vi "Scripting_ChangeBaseClassInSubClass.vi"(0 "SubClass":refnum<vi>, 1 "NewBaseClass":path=path "C:/Projects/Base2_class/Base2.lvclass", 2 "GOOP4Style":bool, 5 "error in (no error)":errorcluster) -> (19 "error out":errorcluster={"status"=TRUE, "code"=1055, "source"="Property Node in Scripting_ConvertBaseClassToSubClass.vi"})   [LabVIEW 2012]
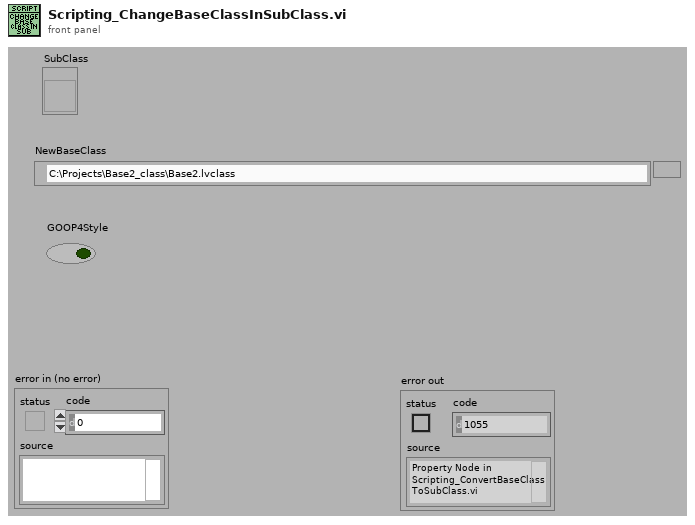
[diagram p1: front panel]
types:
  T1 = cluster{"NewBaseClass":refnum<vi>, "NewBaseClassPath":path, "SubClass":refnum<vi>, "NewBaseClassName":string, "AllBaseClassFiles":path[], "ClassVIs":refnum<vi>[], "CurrentBaseClassRef":refnum<vi>, "CurrentBaseClassPath":path, "CurrentRootBaseClassPath":path, "NewRootBaseClassPath":path}
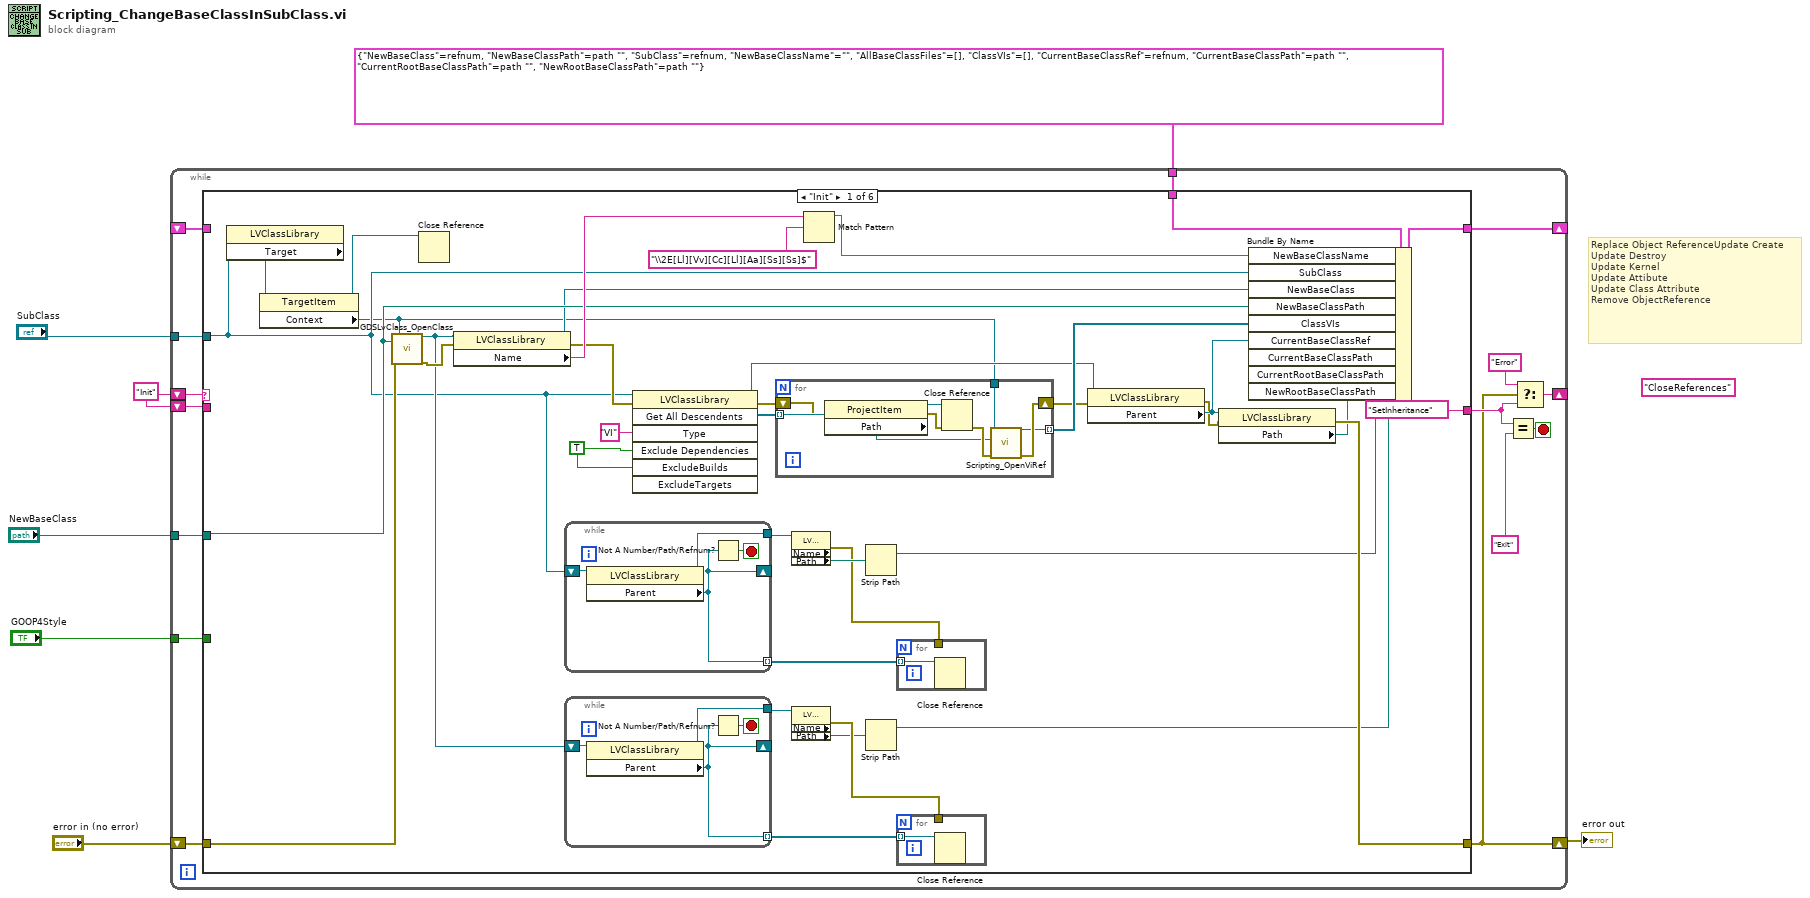
[diagram p0: block diagram]
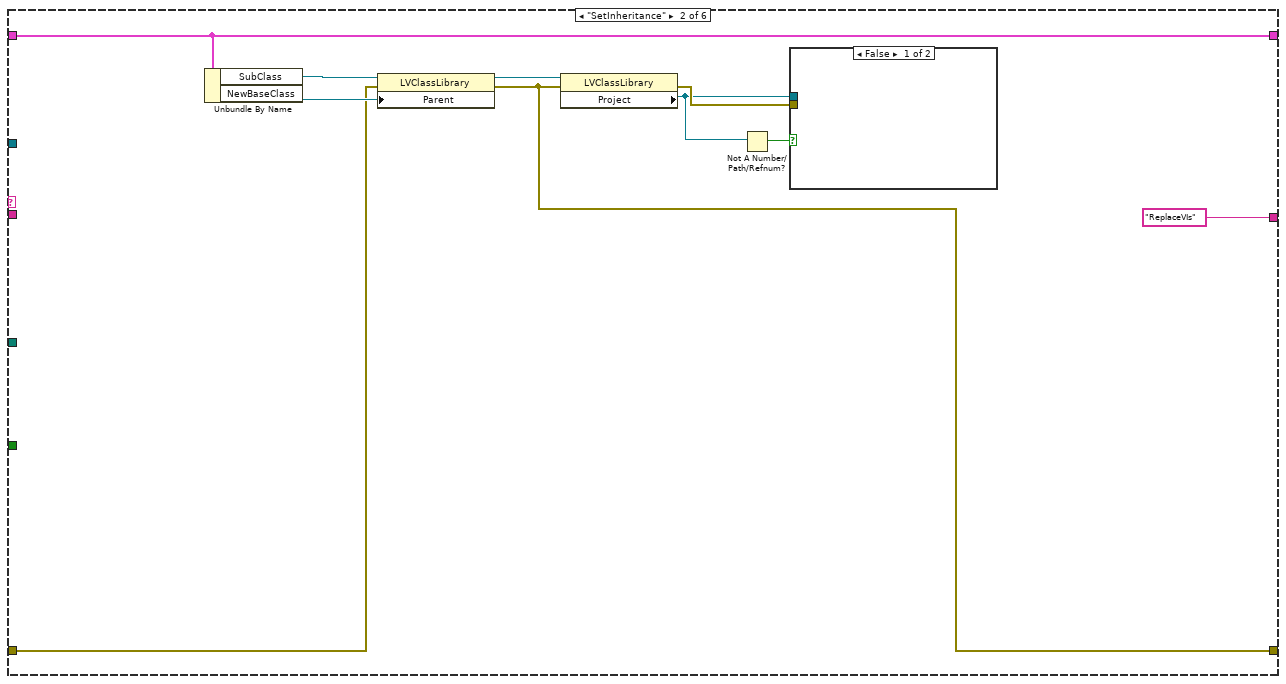
[diagram p2: hidden frame]
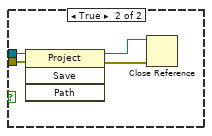
[diagram p3: hidden frame]
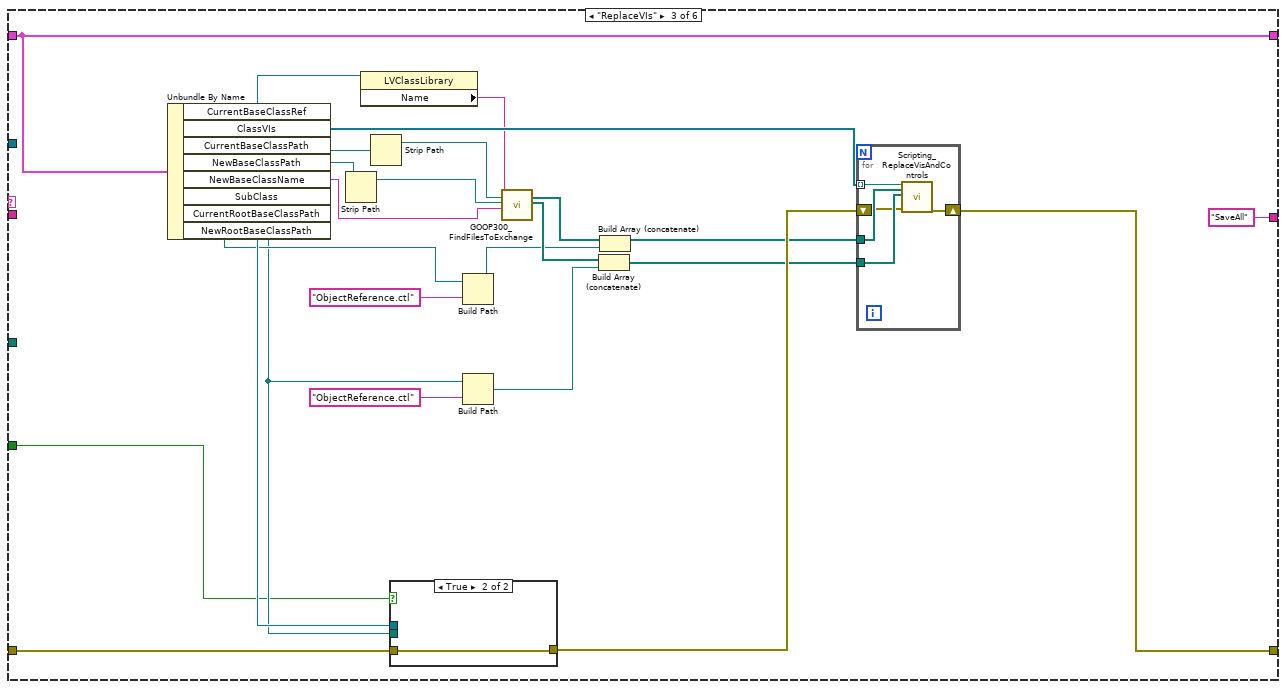
[diagram p4: hidden frame]
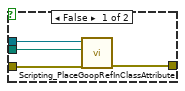
[diagram p5: hidden frame]
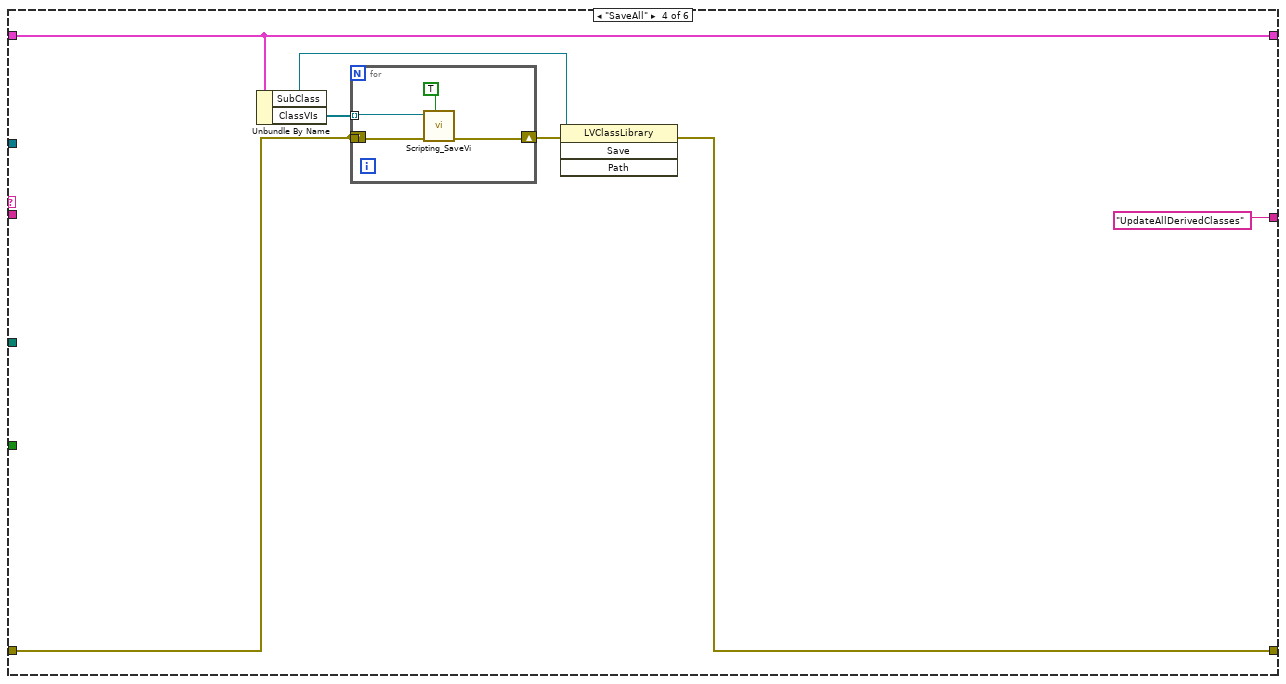
[diagram p6: hidden frame]
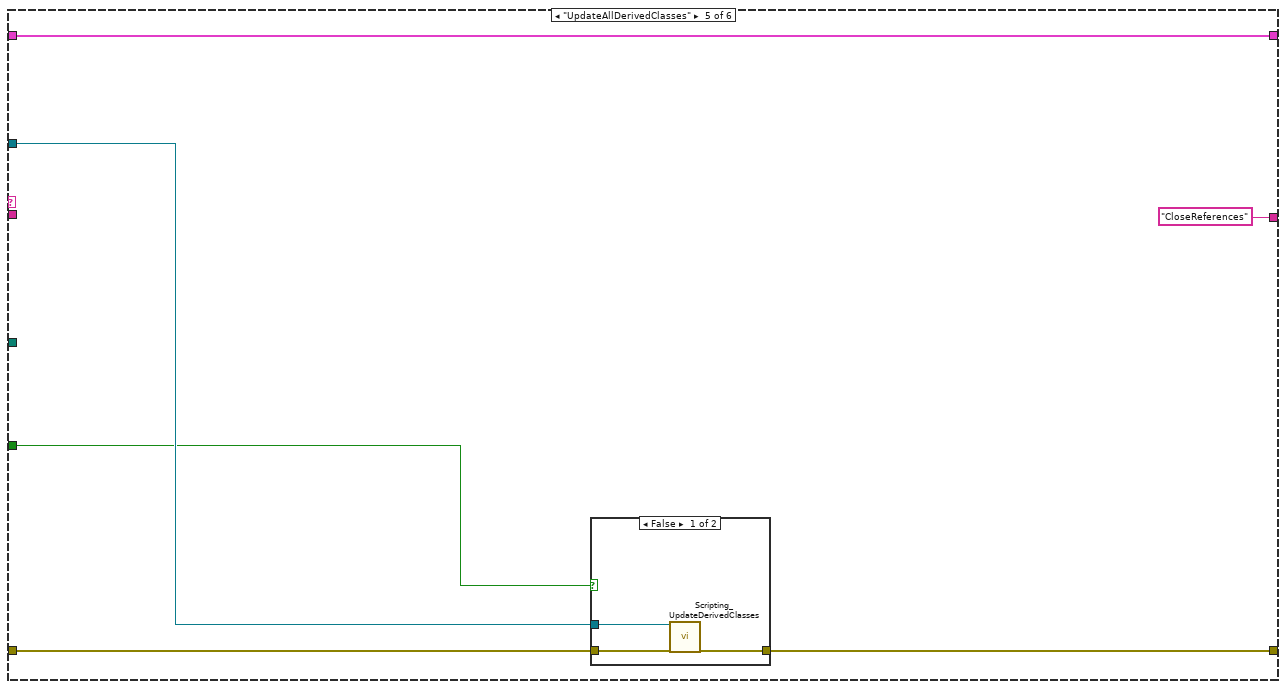
[diagram p7: hidden frame]
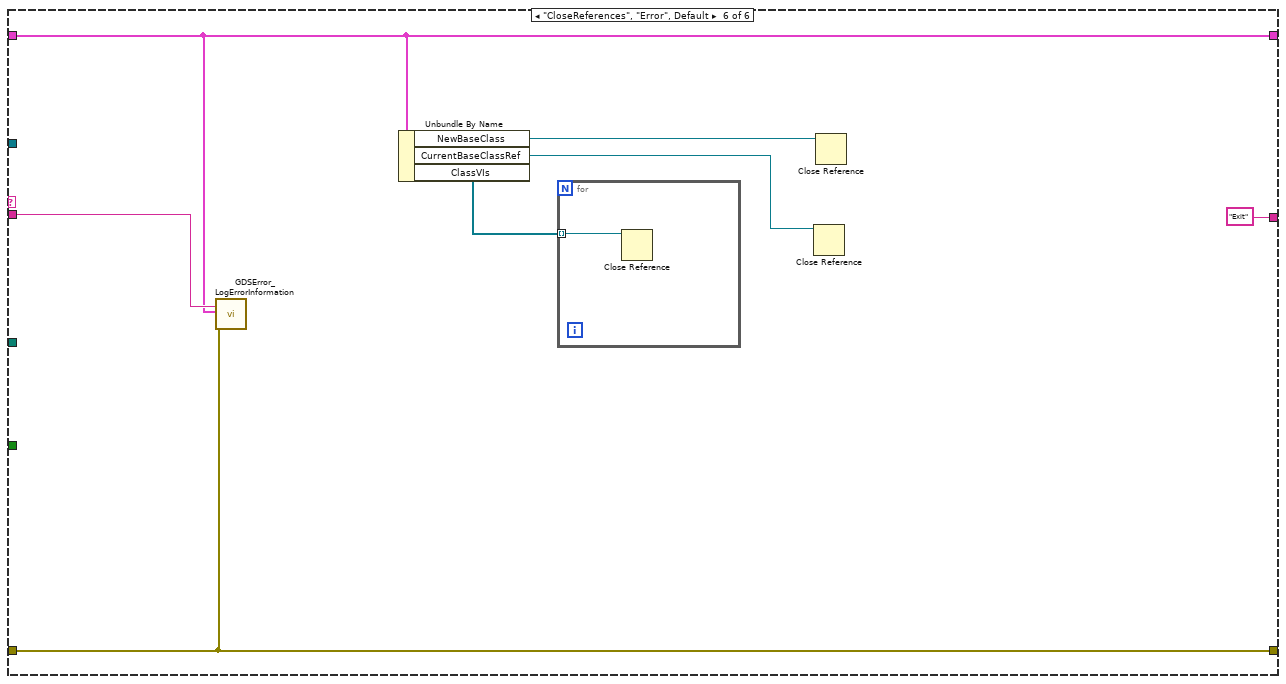
[diagram p9: hidden frame]
diagram:
  (unwired) "CloseReferences"
  w2 = "Init"
  # "Replace Object ReferenceUpdate Create\nUpdate Destroy\nUpdate Kernel\nUpdate Attibute\nUpdate Class Attribute\nRemove ObjectReference"
  n1 = while {
    shift-right: [w15] -> w6
    shift-left: "error in (no error)" -> [w22]
    shift-right: [w20] -> _
    shift-left: w2 -> [w21]
    shift-right: [w14] -> _
    shift-left: _ -> [w13]
    tunnel: "SubClass" -> [w12]
    tunnel: T1 {"NewBaseClass"=refnum, "NewBaseClassPath"=path "", "SubClass"=refnum, "NewBaseClassName"="", "AllBaseClassFiles"=[], "ClassVIs"=[], "CurrentBaseClassRef"=refnum, "CurrentBaseClassPath"=path "", "CurrentRootBaseClassPath"=path "", "NewRootBaseClassPath"=path ""} -> [w11]
    tunnel: "NewBaseClass" -> [w10]
    shift-left: w2 -> [w9]
    tunnel: "GOOP4Style" -> [w8]
    stop <- w19 stop-if-true
    n2 = case shown="\"Init\"" w21 {
      tunnel: w22 -> [w41 w85 w108 w132 w142 w151]
      tunnel: [w49 w79 w116 w129 w140 w151] -> w15
      tunnel: ["SetInheritance" "ReplaceVIs" "SaveAll" "UpdateAllDerivedClasses" "CloseReferences" "Exit"] -> w16
      tunnel: [w59 w87 w112 w133 w143 w149] -> w14
      tunnel: w13 -> [_ w87 w112 w133 w143 w149]
      tunnel: w12 -> [w26 _ _ _ w141 _]
      tunnel: w11 -> [w56 _ _ _ _ _]
      tunnel: w10 -> [w46 _ _ _ _ _]
      tunnel: w9 -> [_ _ _ _ _ w150]
      tunnel: w8 -> [_ _ w93 _ w139 _]
      frame "Init" {
        w27 = TRUE ("ExcludeDependencies")
        n3 = property class="LVClassLibrary"(reference=w26) -> ("Target"=w25:refnum<vi>)  [unwired: 1 in, 2 out]
        n4 = property class="TargetItem"(reference=w25) -> (reference out=w24:refnum<vi>, "Context"=w23:refnum<vi>)  [unwired: 1 in, 1 out]
        n5 = call <resource>:"GDSLvClass_OpenClass.vi"("ClassToOpen"=w46, "error in (no error)"=w41, "Project/ApplicationRef(If empty, currect active project will be used)"=w23) -> ("LVClass.Open"=w29:refnum<vi>, "error out"=w42:errorcluster)  [unwired: 15 in]
        n6 = Close Reference(reference=w24) -> ()  [unwired: 1 in, 1 out]
        n7 = property class="LVClassLibrary"(reference=w29, error in=w42) -> (reference out=w39:refnum<vi>, error out=w40:errorcluster, "Name"=w54:string)
        n8 = while {
          shift-right: [w67] -> _
          shift-left: w26 -> [w68]
          tunnel: [w67] -> w38 mode=indexing
          tunnel: [w66] -> w37
          stop <- w69 stop-if-true
          n9 = property class="LVClassLibrary"(reference=w68) -> (reference out=w66:refnum<vi>, "Parent"=w67:refnum<vi>)  [unwired: 1 in, 1 out]
          n10 = Not A Number/Path/Refnum?(number/path/refnum=w67) -> (NaN/Path/Refnum?=w69:bool)
        }
        n11 = while {
          shift-right: [w62] -> _
          shift-left: w29 -> [w63]
          tunnel: [w62] -> w30 mode=indexing
          tunnel: [w61] -> w31
          stop <- w64 stop-if-true
          n12 = property class="LVClassLibrary"(reference=w63) -> (reference out=w61:refnum<vi>, "Parent"=w62:refnum<vi>)  [unwired: 1 in, 1 out]
          n13 = Not A Number/Path/Refnum?(number/path/refnum=w62) -> (NaN/Path/Refnum?=w64:bool)
        }
        n14 = invoke class="LVClassLibrary" method="Get All Descendents"(reference=w26, error in=w40, "Type"="VI", "Exclude Dependencies"=w27, "ExcludeBuilds"=w27) -> (reference out=w45:refnum<vi>, error out=w57:errorcluster, "All Descendents"=w58:refnum<vi>[])  [unwired: 2 in, 4 out]
        n15 = for {
          tunnel: w58 -> [w78] mode=indexing
          shift-right: [w73] -> w50
          shift-left: w57 -> [w75]
          tunnel: [w71] -> w51 mode=indexing
          tunnel: w23 -> [w70]
          n16 = property class="ProjectItem"(reference=w78, error in=w75) -> (reference out=w77:refnum<vi>, error out=w76:errorcluster, "Path"=w72:path)
          n17 = Close Reference(reference=w77, error in (no error)=w76) -> (error out=w74:errorcluster)
          n18 = call <resource>:"Scripting_OpenViRef.vi"("error in"=w74, "ViPath/ViName"=w72, "AppRef"=w70) -> ("error out"=w73:errorcluster, "vi reference"=w71:refnum<vi>)  [unwired: 7 in]
        }
        n19 = property class="LVClassLibrary" props=["Name", "Path"](reference=w37) -> (error out=w35:errorcluster, "Path"=w36:path)  [unwired: 1 in, 2 out]
        n20 = property class="LVClassLibrary" props=["Name", "Path"](reference=w31) -> (error out=w33:errorcluster, "Path"=w32:path)  [unwired: 1 in, 2 out]
        n21 = Match Pattern(string=w54, regular expression="\\2E[Ll][Vv][Cc][Ll][Aa][Ss][Ss]$") -> (before substring=w53:string)  [unwired: 1 in, 3 out]
        n22 = Strip Path(path=w36) -> (stripped path=w34:path)  [unwired: 1 out]
        n23 = Strip Path(path=w32) -> (stripped path=w28:path)  [unwired: 1 out]
        n24 = for {
          tunnel: w38 -> [w65] mode=indexing
          tunnel: w35 -> [_]
          n25 = Close Reference(reference=w65) -> ()  [unwired: 1 in, 1 out]
        }
        n26 = for {
          tunnel: w30 -> [w60] mode=indexing
          tunnel: w33 -> [_]
          n27 = Close Reference(reference=w60) -> ()  [unwired: 1 in, 1 out]
        }
        n28 = property class="LVClassLibrary"(reference=w45, error in=w50) -> (error out=w44:errorcluster, "Parent"=w48:refnum<vi>)  [unwired: 1 out]
        n29 = property class="LVClassLibrary"(reference=w48, error in=w44) -> (error out=w49:errorcluster, "Path"=w47:path)  [unwired: 1 out]
        n30 = Bundle By Name(cluster=w56, "NewBaseClassName"=w53, "SubClass"=w26, "NewBaseClass"=w39, "NewBaseClassPath"=w46, "ClassVIs"=w51, "CurrentBaseClassRef"=w48, "CurrentBaseClassPath"=w47, "CurrentRootBaseClassPath"=w34, "NewRootBaseClassPath"=w28) -> (w59:T1)
      }
      frame "SetInheritance" {
        n31 = Unbundle By Name(w87) -> ("SubClass"=w88:refnum<vi>, "NewBaseClass"=w86:refnum<vi>)
        n32 = property class="LVClassLibrary"(reference=w88, error in=w85, "Parent"=w86) -> (reference out=w83:refnum<vi>, error out=w79:errorcluster)
        n33 = property class="LVClassLibrary"(reference=w83, error in=w79) -> (error out=w82:errorcluster, "Project"=w81:refnum<vi>)  [unwired: 1 out]
        n34 = Not A Number/Path/Refnum?(number/path/refnum=w81) -> (NaN/Path/Refnum?=w80:bool)
        n35 = case shown="False" w80 {
          tunnel: w82 -> [_ w90]
          tunnel: w81 -> [_ w89]
          frame False {
          }
          frame True {
            n36 = invoke class="Project" method="Save"(reference=w89, error in=w90) -> (reference out=w91:refnum<vi>, error out=w92:errorcluster)  [unwired: 2 in, 2 out]
            n37 = Close Reference(reference=w91, error in (no error)=w92) -> ()  [unwired: 1 out]
          }
        }
      }
      frame "ReplaceVIs" {
        n38 = Unbundle By Name(w112) -> ("CurrentBaseClassRef"=w96:refnum<vi>, "ClassVIs"=w111:refnum<vi>[], "CurrentBaseClassPath"=w115:path, "NewBaseClassPath"=w114:path, "NewBaseClassName"=w94:string, "SubClass"=w109:refnum<vi>, "CurrentRootBaseClassPath"=w101:path, "NewRootBaseClassPath"=w97:path)
        n39 = Strip Path(path=w114) -> (stripped path=w106:path)  [unwired: 1 out]
        n40 = property class="LVClassLibrary"(reference=w96) -> ("Name"=w95:string)  [unwired: 1 in, 2 out]
        n41 = Strip Path(path=w115) -> (stripped path=w110:path)  [unwired: 1 out]
        n42 = case shown="True" w93 {
          tunnel: w109 -> [w121 _]
          tunnel: w108 -> [w120 w122]
          tunnel: [w119 w122] -> w107
          tunnel: w97 -> [w118 _]
          frame False {
            n43 = call <resource>:"Scripting_PlaceGoopRefInClassAttribute.vi"("error in"=w120, "ObjectRef_LvClassFolderPath"=w118, "ClassRefnum"=w121) -> ("error out"=w119:errorcluster)  [unwired: 1 in, 3 out]
          }
          frame True {
          }
        }
        n44 = Build Path(base path=w101, name or relative path="ObjectReference.ctl" ("element")) -> (appended path=w100:path)
        n45 = Build Path(base path=w97, name or relative path="ObjectReference.ctl" ("element")) -> (appended path=w98:path)
        n46 = call <resource>:"GOOP300_FindFilesToExchange.vi"("OldClassName(Prefix or suffix for some VIs)"=w95, "OldFolderPath"=w110, "NewFolderPath"=w106, "NewClassName(Prefix or suffix for some VIs)"=w94) -> ("OldFiles"=w113:path[], "NewFileArray"=w104:path[])  [unwired: 14 in]
        n47 = Build Array (concatenate)(w104, w98) -> (w103:path[])
        n48 = Build Array (concatenate)(w113, w100) -> (w105:path[])
        n49 = for {
          shift-right: [w127] -> w116
          shift-left: w107 -> [w124]
          tunnel: w105 -> [w126]
          tunnel: w103 -> [w125]
          tunnel: w111 -> [w123] mode=indexing
          n50 = call <resource>:"Scripting_ReplaceVisAndControls.vi"("ViRef"=w123, "OldVIsAndControls"=w126, "NewVIsAndControls"=w125, "error in (no error)"=w124) -> ("error out"=w127:errorcluster)  [unwired: 14 in, 1 out]
        }
      }
      frame "SaveAll" {
        n51 = Unbundle By Name(w133) -> ("SubClass"=w130:refnum<vi>, "ClassVIs"=w134:refnum<vi>[])
        n52 = for {
          tunnel: w134 -> [w138] mode=indexing
          shift-right: [w135] -> w131
          shift-left: w132 -> [_]
          tunnel: w132 -> [w136]
          n53 = call <resource>:"Scripting_SaveVi.vi"("ForceResaving(False)"=TRUE, "error in (no error)"=w136, "VIRefToSaveIn"=w138) -> ("error out"=w135:errorcluster)  [unwired: 7 in, 1 out]
        }
        n54 = invoke class="LVClassLibrary" method="Save"(reference=w130, error in=w131) -> (error out=w129:errorcluster)  [unwired: 2 in, 3 out]
      }
      frame "UpdateAllDerivedClasses" {
        n55 = case shown="False" w139 {
          tunnel: w142 -> [w147 w148]
          tunnel: w141 -> [w146 _]
          tunnel: [w145 w148] -> w140
          frame False {
            n56 = call <resource>:"Scripting_UpdateDerivedClasses.vi"("ClassRef"=w146, "error in (no error)"=w147) -> ("error out"=w145:errorcluster)  [unwired: 17 in]
          }
          frame True {
          }
        }
      }
      frame "CloseReferences", "Error", Default {
        n57 = call <resource>:"GDSError_LogErrorInformation.vi"("State"=w150, "LocalVariableData"=w149, "error in (no error)"=w151) -> ()  [unwired: 16 in, 1 out]
        n58 = Unbundle By Name(w149) -> ("NewBaseClass"=w155:refnum<vi>, "CurrentBaseClassRef"=w153:refnum<vi>, "ClassVIs"=w152:refnum<vi>[])
        n59 = for {
          tunnel: w152 -> [w156] mode=indexing
          n60 = Close Reference(reference=w156) -> ()  [unwired: 1 in, 1 out]
        }
        n61 = Close Reference(reference=w153) -> ()  [unwired: 1 in, 1 out]
        n62 = Close Reference(reference=w155) -> ()  [unwired: 1 in, 1 out]
      }
    }
    n63 = Equal?(x=w16, y="Exit") -> (x = y?=w19:bool)
    n64 = Select(t="Error", s=w15, f=w16) -> (s? t:f=w20:string)
  }
  "error out" <- w6
